vi "llenado_timer.vi"() -> ()   [LabVIEW 2022 SP3]
uses:
  <vilib>/Instr/_visa.llb/VISA Configure Serial Port (Instr).vi
panel:
  in  "DEBUG":string
  out "slide":dbl(slide) scale=0.0..500.0
  in  "contenedor":dbl(slide) scale=0.0..10.0
  out "Slide 2":u8(slide) scale=0.0..100.0
  out "Slide":u8(slide) scale=0.0..100.0
  out "valvula":bool
  out "bomba":bool
  out "e_valvula":bool
  out "e_bomba":bool
  in  "btn_stop":bool
  in  "btn_cancelar":bool
  in  "btn_iniciar":bool
  out "s_nivel":bool
  in  "VISA resource name":refnum<visa-resource-name>
  out "Slide 3":u8(slide) scale=0.0..100.0
  # "Puerto del Microcontroaldor"
  # "Control de llenado"
  # "Iniciar secuencia de llenado"
  # "Cancelar secuencia de llenado"
  # "Detener ejecucion de programa"
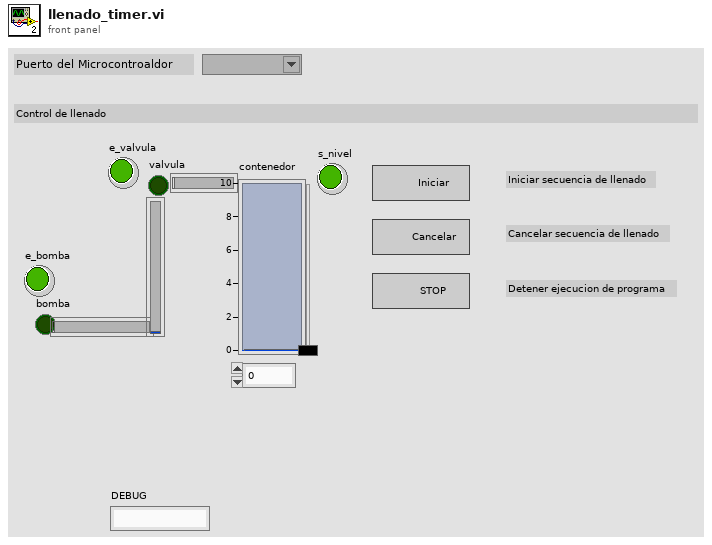
[diagram p1: front panel]
types:
  T1 = enum16{"init", "idle", "filling", "pause", "stop"}
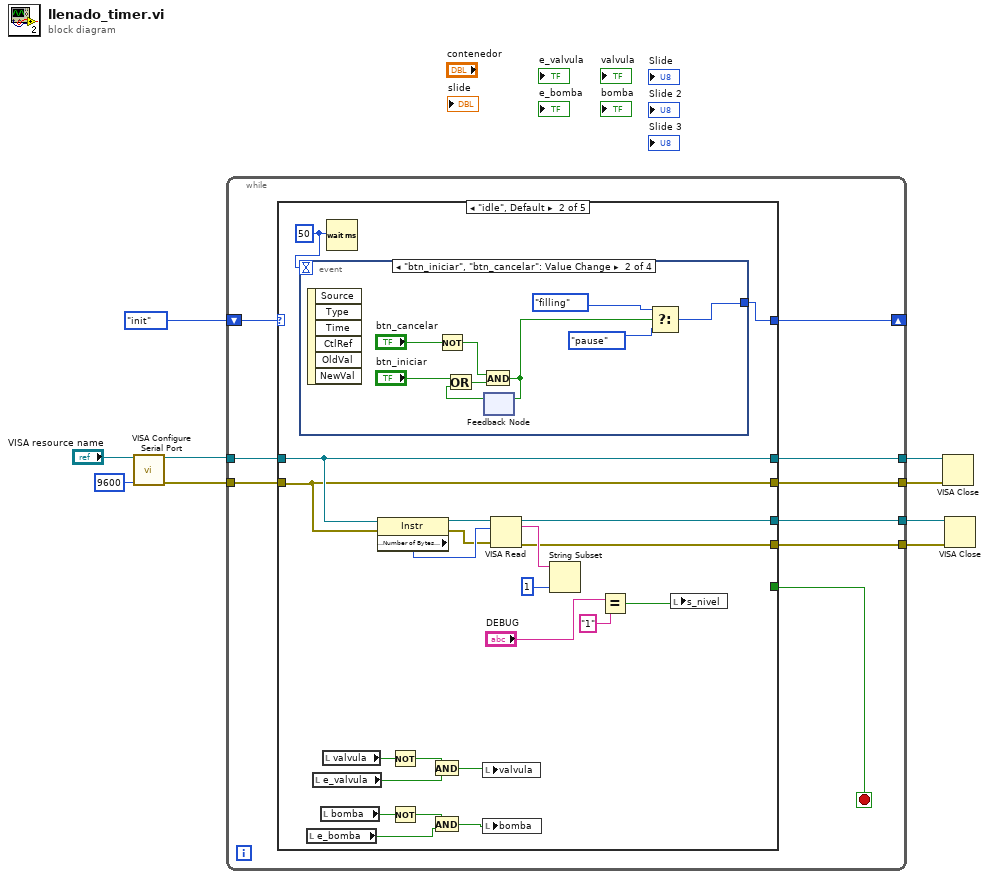
[diagram p0: block diagram]
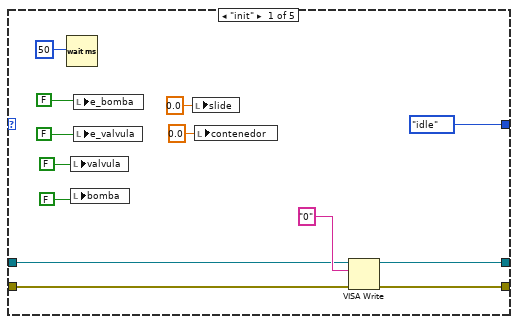
[diagram p2: hidden frame]
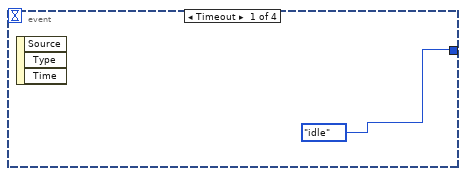
[diagram p3: hidden frame]
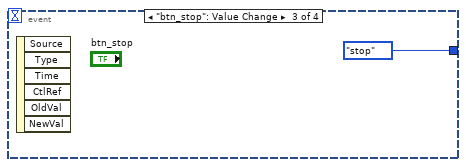
[diagram p4: hidden frame]
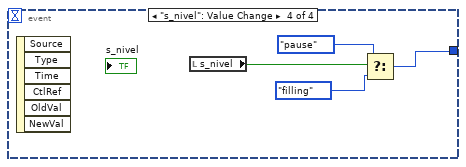
[diagram p5: hidden frame]
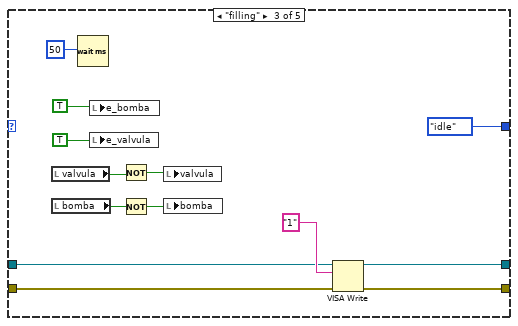
[diagram p6: hidden frame]
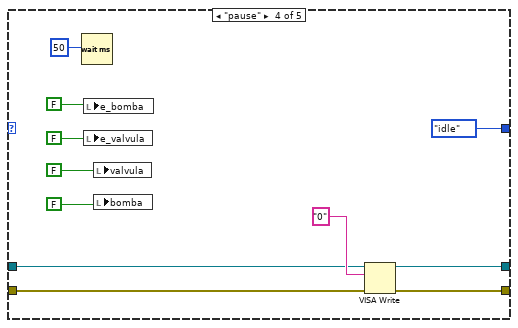
[diagram p7: hidden frame]
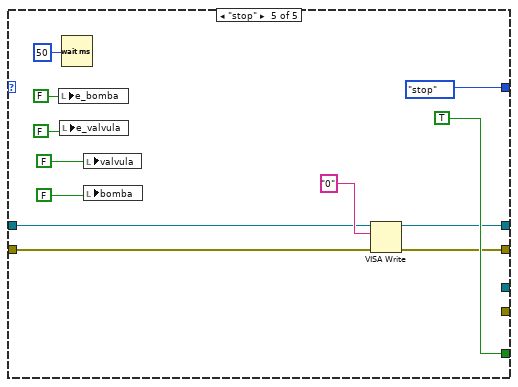
[diagram p8: hidden frame]
diagram:
  n1 = call-poly "VISA Configure Serial Port"("VISA resource name"="VISA resource name", "baud rate (9600)"=u32 9600) -> ("VISA resource name out"=w7:refnum<visa-resource-name>, "error out"=w6:errorcluster)  [unwired: 12 in]
  n2 = while {
    tunnel: [w10] -> w5
    tunnel: [w11] -> w4
    shift-right: [w17] -> _
    shift-left: T1."init" -> [w18]
    tunnel: w6 -> [w14]
    tunnel: w7 -> [w15]
    tunnel: [w12] -> w2
    tunnel: [w13] -> w1
    stop <- w16 stop-if-true
    n3 = case shown="\"idle\", Default" w18 {
      tunnel: [T1."idle" w52 T1."idle" T1."idle" T1."stop"] -> w17
      tunnel: [_ _ _ _ TRUE] -> w16
      tunnel: w15 -> [w24 w39 w80 w91 w98]
      tunnel: w14 -> [w23 w38 w79 w89 w97]
      tunnel: [w22 w38 w77 w88 w95] -> w13
      tunnel: [w21 w39 w78 w90 w96] -> w12
      tunnel: [_ w37 _ _ _] -> w11
      tunnel: [_ w36 _ _ _] -> w10
      frame "init" {
        n4 = Wait (ms)(milliseconds to wait=50) -> ()  [unwired: 1 out]
        n5 = local write "valvula"(FALSE) -> ()
        n6 = local write "bomba"(FALSE) -> ()
        n7 = local write "e_bomba"(FALSE) -> ()
        n8 = local write "e_valvula"(FALSE) -> ()
        n9 = local write "slide"(0.0 ("slide")) -> ()
        n10 = local write "contenedor"(0.0 ("contenedor")) -> ()
        n11 = VISA Write(VISA resource name=w24, write buffer="0", error in (no error)=w23) -> (VISA resource name out=w21:refnum<visa-resource-name>, error out=w22:errorcluster)  [unwired: 1 out]
      }
      frame "idle", Default {
        w53 = 50
        n12 = event shown="[1] \"btn_iniciar\", \"btn_cancelar\": Value Change" {
          selector: _ -> [_ _ _ _]
          dyn-events: _ -> [_ _ _ _]
          timeout: w53 -> [_ _ _ _]
          tunnel: [T1."idle" w59 T1."stop" w68] -> w52
          event Timeout {
            n13 = event-data() -> ()  [unwired: 1 in, 3 out]
          }
          event "btn_iniciar", "btn_cancelar": Value Change {
            n14 = event-data() -> ()  [unwired: 1 in, 6 out]
            n15 = Not(x="btn_cancelar") -> (.not. x?=w63:bool)
            n16 = feedback #1() -> (w61:bool)  [unwired: 1 in]
            n17 = Or(x="btn_iniciar", y=w61) -> (x .or. y?=w62:bool)
            n18 = And(x=w63, y=w62) -> (x .and. y?=w60:bool)
            n19 = feedback-in #1(w60) -> ()
            n20 = Select(t=T1."filling", s=w60, f=T1."pause") -> (s? t:f=w59:T1)
          }
          event "btn_stop": Value Change {
            n21 = event-data() -> ()  [unwired: 1 in, 6 out]
          }
          event "s_nivel": Value Change {
            n22 = event-data() -> ()  [unwired: 1 in, 6 out]
            n23 = local read "s_nivel"() -> (w65:bool)
            n24 = Select(t=T1."pause", s=w65, f=T1."filling") -> (s? t:f=w68:T1)
          }
        }
        n25 = local read "e_bomba"() -> (w44:bool)
        n26 = local read "e_valvula"() -> (w48:bool)
        n27 = local read "bomba"() -> (w45:bool)
        n28 = local read "valvula"() -> (w51:bool)
        n29 = Wait (ms)(milliseconds to wait=w53) -> ()  [unwired: 1 out]
        n30 = property class="Instr"(reference=w39, error in=w38) -> (reference out=w40:refnum<visa-resource-name>, error out=w41:errorcluster, "Serial Settings:Number of Bytes at Serial Port"=w42:u32)
        n31 = Not(x=w51) -> (.not. x?=w50:bool)
        n32 = Not(x=w45) -> (.not. x?=w47:bool)
        n33 = And(x=w50, y=w48) -> (x .and. y?=w49:bool)
        n34 = And(x=w47, y=w44) -> (x .and. y?=w46:bool)
        n35 = local write "valvula"(w49) -> ()
        n36 = local write "bomba"(w46) -> ()
        n37 = VISA Read(VISA resource name=w40, byte count=w42, error in (no error)=w41) -> (VISA resource name out=w36:refnum<visa-resource-name>, read buffer=w43:string, error out=w37:errorcluster)  [unwired: 1 out]
        n38 = String Subset(string=w43, length (rest)=1) -> ()  [unwired: 1 in, 1 out]
        n39 = Equal?(x="DEBUG", y="1") -> (x = y?=w32:bool)
        n40 = local write "s_nivel"(w32) -> ()
      }
      frame "filling" {
        n41 = local read "valvula"() -> (w74:bool)
        n42 = local read "bomba"() -> (w73:bool)
        n43 = Wait (ms)(milliseconds to wait=50) -> ()  [unwired: 1 out]
        n44 = local write "e_bomba"(TRUE) -> ()
        n45 = local write "e_valvula"(TRUE) -> ()
        n46 = Not(x=w74) -> (.not. x?=w71:bool)
        n47 = Not(x=w73) -> (.not. x?=w72:bool)
        n48 = local write "valvula"(w71) -> ()
        n49 = local write "bomba"(w72) -> ()
        n50 = VISA Write(VISA resource name=w80, write buffer="1", error in (no error)=w79) -> (VISA resource name out=w78:refnum<visa-resource-name>, error out=w77:errorcluster)  [unwired: 1 out]
      }
      frame "pause" {
        n51 = Wait (ms)(milliseconds to wait=50) -> ()  [unwired: 1 out]
        n52 = local write "e_bomba"(FALSE) -> ()
        n53 = local write "e_valvula"(FALSE) -> ()
        n54 = local write "valvula"(FALSE) -> ()
        n55 = local write "bomba"(FALSE) -> ()
        n56 = VISA Write(VISA resource name=w91, write buffer="0", error in (no error)=w89) -> (VISA resource name out=w90:refnum<visa-resource-name>, error out=w88:errorcluster)  [unwired: 1 out]
      }
      frame "stop" {
        n57 = local write "e_bomba"(FALSE) -> ()
        n58 = local write "e_valvula"(FALSE) -> ()
        n59 = Wait (ms)(milliseconds to wait=50) -> ()  [unwired: 1 out]
        n60 = local write "valvula"(FALSE) -> ()
        n61 = local write "bomba"(FALSE) -> ()
        n62 = VISA Write(VISA resource name=w98, write buffer="0", error in (no error)=w97) -> (VISA resource name out=w96:refnum<visa-resource-name>, error out=w95:errorcluster)  [unwired: 1 out]
      }
    }
  }
  n63 = VISA Close(VISA resource name=w2, error in (no error)=w1) -> ()  [unwired: 1 out]
  n64 = VISA Close(VISA resource name=w5, error in (no error)=w4) -> ()  [unwired: 1 out]
